vi "Position Circumnavigate radius slider.vi"(8 "error in (no error)":errorcluster, 10 "Upper Slider":refnum<vi>, 11 "DigNum Refnum":refnum<vi>) -> (0 "error out":errorcluster)   [LabVIEW 2014]
panel:
  in  "Desired Altitude (m)":dbl=20.0 step=1.0
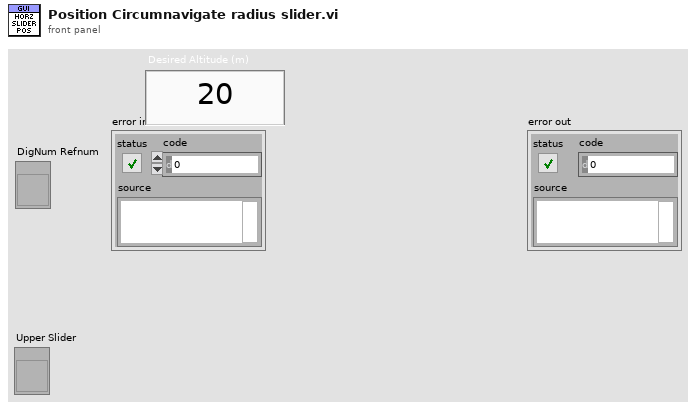
[diagram p1: front panel]
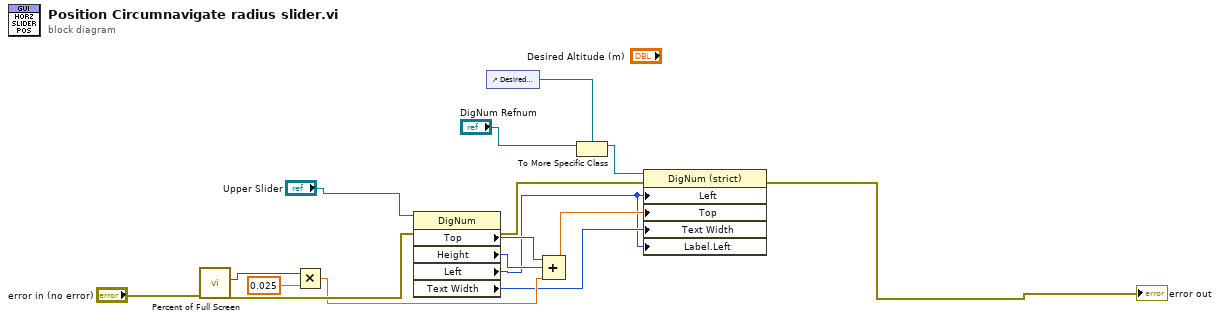
[diagram p0: block diagram]
diagram:
  n1 = call "Percent of Full Screen.vi"("error in (no error)"="error in (no error)") -> ("error out"=w12:errorcluster, "Bottom"=w9:i16)  [unwired: 8 in, 1 out]
  n2 = Multiply(x=w9, y=0.025) -> (x*y=w7:dbl)
  n3 = property class="DigNum"(reference="Upper Slider", error in=w12) -> (error out=w13:errorcluster, "Top"=w15:i32, "Height"=w14:u32, "Left"=w1:i32, "Text Width"=w2:u32)  [unwired: 1 out]
  n4 = control-ref of="Desired Altitude (m)"() -> (w5:refnum<vi>)
  n5 = Compound Arithmetic op=ADD(w15, w14, w7) -> (w10:dbl)
  n6 = To More Specific Class(target class=w5, reference="DigNum Refnum") -> (specific class reference=w4:refnum<vi>)  [unwired: 1 in, 1 out]
  n7 = property class="DigNum (strict)"(reference=w4, error in=w13, "Left"=w1, "Top"=w10, "Text Width"=w2, "Label.Left"=w1) -> (error out=→"error out":errorcluster)  [unwired: 1 out]
